vi "acquisition-system-atwood-machine.vi"() -> ()   [LabVIEW 2014]
uses:
  <vilib>/userdefined/High Color/IMAQdx.ctl
  LINX/Digital Write 1 Chan.vi
  <vilib>/MakerHub/LINX/Public/Peripherals/Analog/Analog Read 1 Chan.vi
  <vilib>/MakerHub/LINX/Public/Peripherals/Digital/Digital Write N Chans.vi
  <vilib>/MakerHub/LINX/Public/Peripherals/Analog/Analog Read N Chans.vi
  <vilib>/MakerHub/LINX/Private/Local IO/LinxDigitalWrite.vi
  <vilib>/MakerHub/LINX/Public/Utilities/Check Channel.vi
  <vilib>/MakerHub/LINX/Private/Local IO/LinxAnalogRead.vi
  <vilib>/MakerHub/LINX/Public/Utilities/Open Serial.vi
  <vilib>/MakerHub/LINX/Private/Utilties/Generate Error.vi
  <vilib>/MakerHub/LINX/LMH-LINX.lvlib
  <vilib>/vision/driver/NI_Vision_Acquisition_Software.lvlib
panel:
  in  "?":enum32{"Button", "Data", "Export Data"}(tab)
  in  "OK Button":bool
  out "?":T1(plugin-control)
  in  "CHANNEL WEBCAM":T2
  in  "TABEL PENGAMBILAN DATA":string[][](table)
  out "Time B-C (s)":string[][](table)
  out "Time A-B (s)":string[][](table)
  in  "?":bool
  out "Indicator of IR 1":bool
  out "Indicator of IR 2":bool
  out "Timer 2 (s)":dbl caption="Elapsed Time (s)"
  out "Timer 1 (s)":dbl caption="Elapsed Time (s)"
  # "Data Acquisition System for Atwood Machine Experiment"
  # "Apparatus Scetch"
  # "Camera"
  # "Sensor Indicator"
  # "Data Table"
  # "Experimental Data"
  # "Instructions for use"
  # "Information"
  # "m      = massa beban tambahan \n t_AB  = waktu tempuh beban (M) untuk\n             bergerak dari titik A ke B\n t_BC  = waktu tempuh beban (M) untuk\n             bergerak dari titik B ke C\n M1    = massa beban 1\n M2    = massa beban 2\n S_AB  = jarak dari titik A ke titik B\n S_BC  = jarak dari titik A ke titik B"
  # "Release Button"
  # "© 2021, Physics Education Department"
  # "- Set the webcam channel on the available channels;\n\n- Press RUN to run the system;\n\n- Press the \"RELEASE\" button to start the experiment;\n\n- Press the \"STOP\" button after the experimental data is obtained;"
  # "- The experimental data of AB and BC time will be displayed in their respective tables;\n\n- Time data AB and BC are the numbers/values in the first row listed in each table;\n\n- After the data is obtained, move each data (AB & BC time) to the data retrieval table that is already available"
  # "After completing the experiment, export the data to Microsoft Office\nExcel for further analysis.\n\nBlock all data -> right click -> Export -> export data to excel."
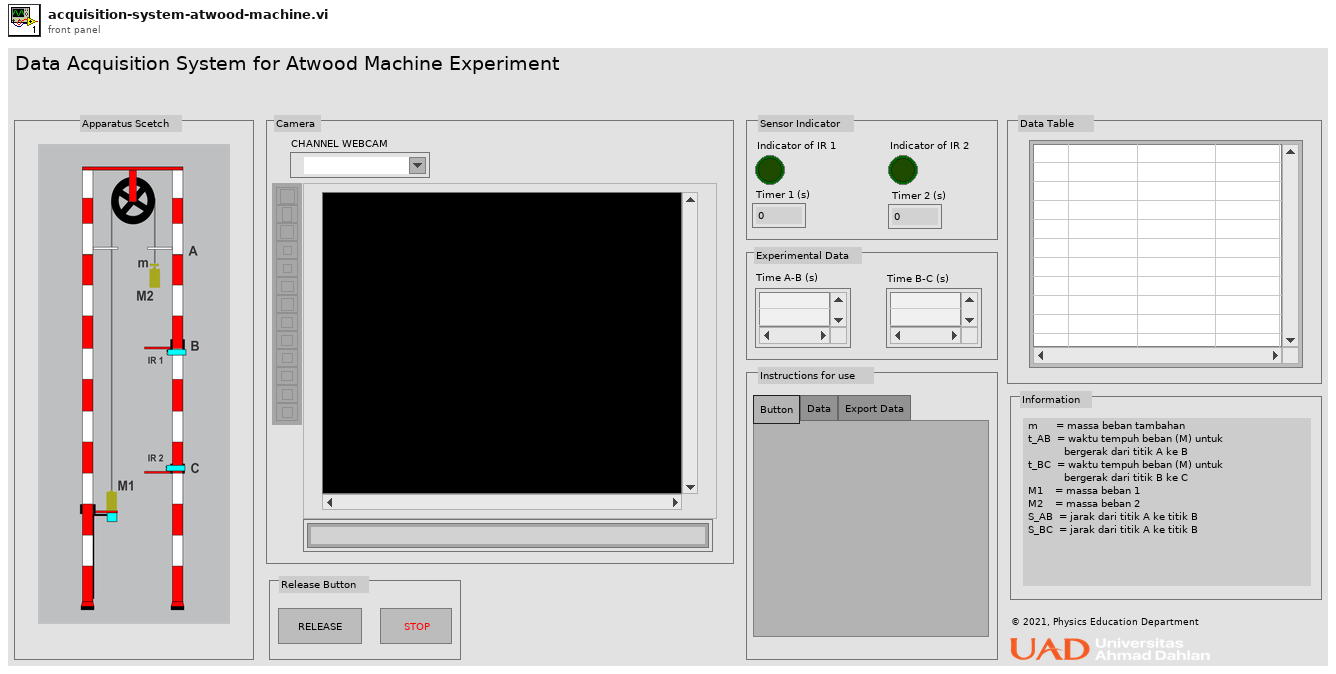
[diagram p1: front panel]
types:
  T1 = typedef "IMAQ Image.ctl" = refnum<image>
  T2 = typedef "IMAQdx.ctl" = refnum<k21>
  T3 = typedef "Image Type" = u32
  T4 = typedef "LMH-LINX.lvlib/LINX Ref.ctl" = cluster{"IO":T5, "Interface":T6, "LINX Device Config":T7}
  T5 = typedef "LMH-LINX.lvlib/Platform.ctl" = enum16{"Remote", "Local"}
  T6 = typedef "LMH-LINX.lvlib/Interface.ctl" = enum16{"Serial", "TCP"}
  T7 = typedef "LMH-LINX.lvlib/Device.lvlib/LINX Device Config.ctl" = cluster{"Interface":T6, "COM Port":refnum<visa-resource-name>, "TCP Configuration":T8, "Device Family":u8, "Device ID":u8, "Device Name":string, "TCP Ref":refnum<k5>, "Channels":T9}
  T8 = typedef "LMH-LINX.lvlib/Device.lvlib/TCP Config.ctl" = cluster{"IP Address":string, "Port":u16}
  T9 = typedef "LMH-LINX.lvlib/Channels.ctl" = cluster{"DI":u8[], "DO":u8[], "AI":u8[], "AO":u8[], "PWM":u8[], "QE":u8[], "UART":u8[], "I2C 2":u8[], "SPI":u8[], "CAN":u8[], "Servo":u8[], "AI Ref (V)":dbl, "AI Resolution (Bits)":u8, "AO Ref (V)":dbl, "AO Resolution (Bits)":u8}
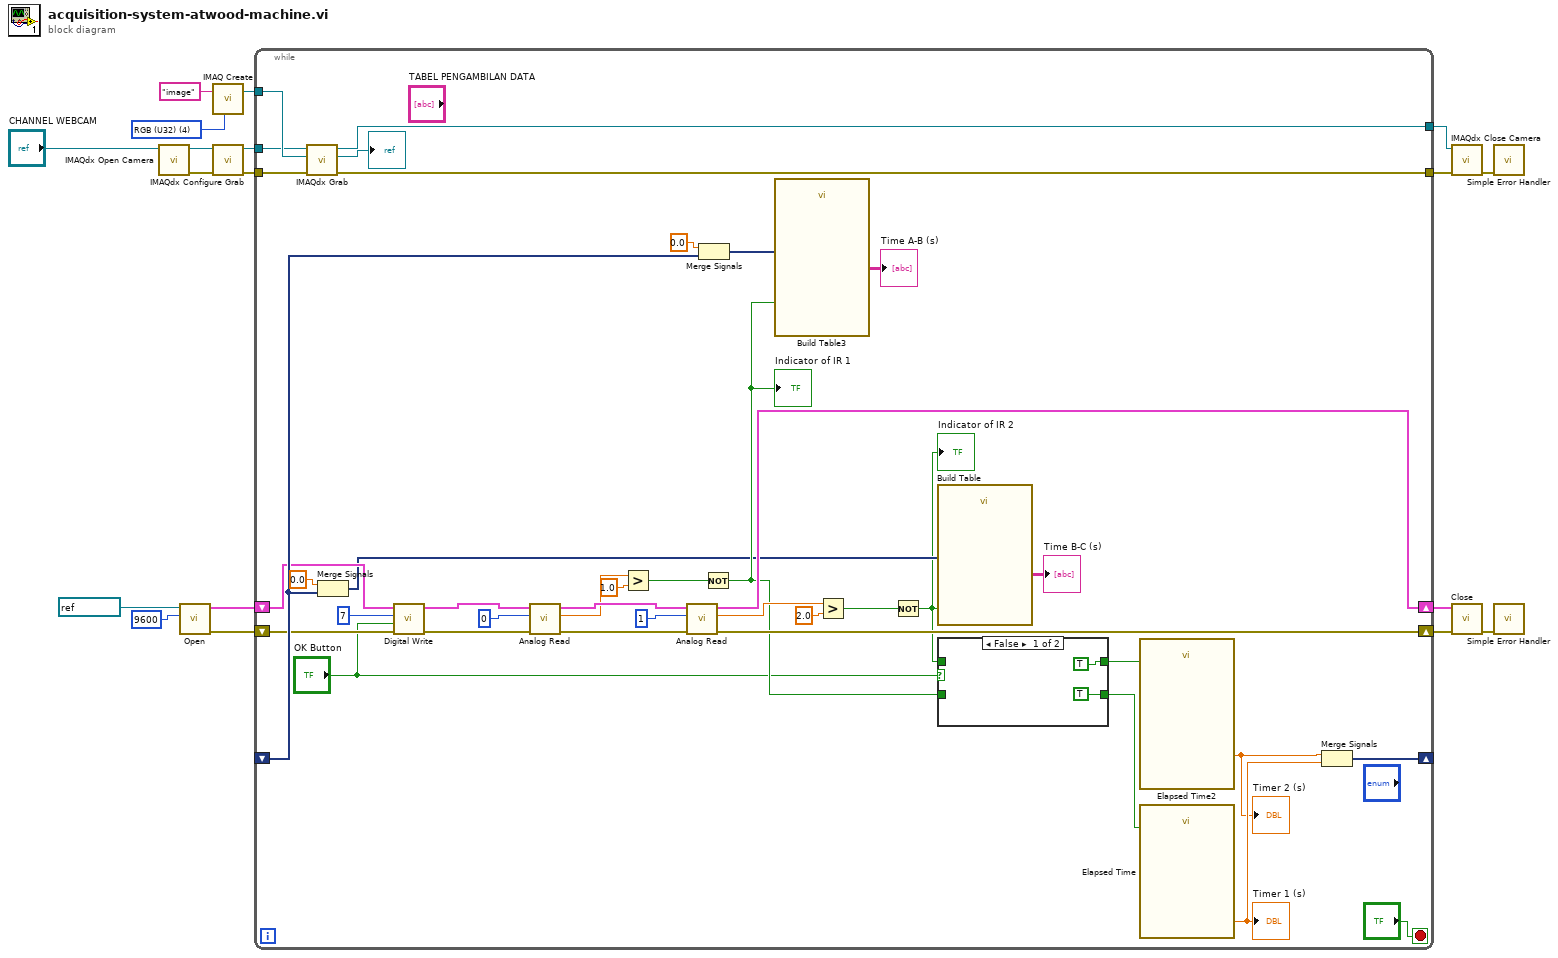
[diagram p0: block diagram]
diagram:
  w5 = T3 4 items=["Grayscale (U8)", "Grayscale (I16)", "Grayscale (SGL)", "Complex (CSG)", "RGB (U32)", "HSL (U32)", "RGB (U64)", "Grayscale (U16)"] ("Image Type")
  n1 = call <vilib>:"IMAQdx Open Camera.vi"("Session In"="CHANNEL WEBCAM") -> ("error out"=w9:errorcluster, "Session Out"=w10:T2)  [unwired: 9 in]
  n2 = call-poly <vilib>:"Open.vi"("Baud Rate Override"=u32 9600, "Serial Port"=refnum<visa-resource-name> "COM3") -> ("Error Out"=w14:errorcluster, "LINX Resource"=w18:T4)  [unwired: 7 in, 1 out]
  n3 = call "IMAQ Create"("Image Name"="image", "Image Type"=w5) -> ("New Image"=w6:T1)  [unwired: 3 in, 1 out]
  n4 = call <vilib>:"IMAQdx Configure Grab.vi"("error in"=w9, "Session In"=w10) -> ("error out"=w7:errorcluster, "Session Out"=w8:T2)  [unwired: 8 in]
  n5 = while {
    shift-right: [w53] -> w17
    shift-left: w18 -> [w43]
    shift-right: [w52] -> w15
    shift-left: w14 -> [w40]
    shift-right: [w46] -> _
    shift-left: _ -> [w47]
    tunnel: w8 -> [w19]
    tunnel: w7 -> [w21]
    tunnel: [w24] -> w3
    tunnel: [w22] -> w2
    tunnel: w6 -> [w20]
    stop <- "?" stop-if-true
    n6 = call <vilib>:"IMAQdx Grab.vi"("error in"=w21, "Image In"=w20, "Session In"=w19) -> ("error out"=w22:errorcluster, "Image Out"=→"?":T1, "Session Out"=w24:T2)  [unwired: 5 in, 1 out]
    n7 = Merge Signals(0.0, w47) -> (w29:dynamicdata)
    n8 = call-poly <vilib>:"Digital Write.vi"("Error In"=w40, "Output Value"="OK Button", "DO Channel"=u8 7, "LINX Resource"=w43) -> ("Error Out"=w41:errorcluster, "LINX Resource"=w42:T4)  [unwired: 6 in]
    n9 = call-poly <vilib>:"Analog Read.vi"("Error In"=w41, "Analog Channel"=u8 0, "LINX Resource"=w42) -> ("Error Out"=w54:errorcluster, "Voltage"=w45:dbl, "LINX Resource"=w55:T4)  [unwired: 5 in, 1 out]
    n10 = Greater?(x=w45, y=1.0) -> (0:w57:bool)
    n11 = call-poly <vilib>:"Analog Read.vi"("Error In"=w54, "Analog Channel"=u8 1, "LINX Resource"=w55) -> ("Error Out"=w52:errorcluster, "Voltage"=w35:dbl, "LINX Resource"=w53:T4)  [unwired: 5 in, 1 out]
    n12 = Merge Signals(0.0, w47) -> (w32:dynamicdata)
    n13 = Not(x=w57) -> (.not. x?=w31:bool)
    "Indicator of IR 1" <- w31
    n14 = call "Build Table3"("Enable"=w31, "Signals"=w32) -> ("Table"=→"Time A-B (s)":string[][])  [unwired: 3 in, 6 out]
    n15 = Greater?(x=w35, y=2.0) -> (0:w50:bool)
    n16 = Not(x=w50) -> (.not. x?=w28:bool)
    "Indicator of IR 2" <- w28
    n17 = call "Build Table"("Enable"=w28, "Signals"=w29) -> ("Table"=→"Time B-C (s)":string[][])  [unwired: 3 in, 6 out]
    n18 = case shown="False" "OK Button" {
      tunnel: w28 -> [_ w61]
      tunnel: [TRUE w61] -> w37
      tunnel: w31 -> [_ w60]
      tunnel: [TRUE w60] -> w36
      frame False {
      }
      frame True {
      }
    }
    n19 = call "Elapsed Time2"("Reset"=w37) -> ("Elapsed Time (s)"=w38:dbl)  [unwired: 11 in, 7 out]
    "Timer 2 (s)" <- w38
    n20 = call "Elapsed Time"("Reset"=w36) -> ("Elapsed Time (s)"=w39:dbl)  [unwired: 11 in, 7 out]
    "Timer 1 (s)" <- w39
    n21 = Merge Signals(w38, w39) -> (w46:dynamicdata)
  }
  n22 = call <vilib>:"IMAQdx Close Camera.vi"("error in"=w2, "Session In"=w3) -> ("error out"=w1:errorcluster)  [unwired: 9 in]
  n23 = call <vilib>:"Close.vi"("Error In"=w15, "LINX Resource"=w17) -> ("Error Out"=w13:errorcluster)  [unwired: 9 in]
  n24 = call <vilib>:"Simple Error Handler.vi"("error in (no error)"=w1) -> ()  [unwired: 4 in, 5 out]
  n25 = call <vilib>:"Simple Error Handler.vi"("error in (no error)"=w13) -> ()  [unwired: 4 in, 5 out]
